vi "Test_WriteValue_InvalidRefnum_Error.vi"(8 "error in (no error)":errorcluster, 11 "TestCase in":refnum<class "TestTerminalSignalingValueBinding.lvclass">) -> (0 "error out":errorcluster, 3 "TestCase out":refnum<class "TestTerminalSignalingValueBinding.lvclass">)   [LabVIEW 2017, in "TestTerminalSignalingValueBinding.lvclass"]
uses:
  TestTerminalSignalingValueBinding.lvclass
  Source/Concrete/TerminalSignalingValueBinding/TerminalSignalingValueBinding.lvclass
  C:/Git/composed-transport/Source/ITransport/ITransport.lvclass
  Source/ITransport/ITransport.lvclass
panel:
  out "Return Error":errorcluster
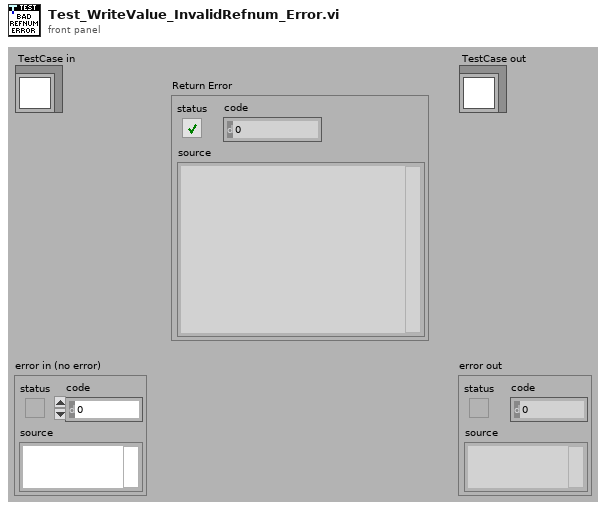
[diagram p1: front panel]
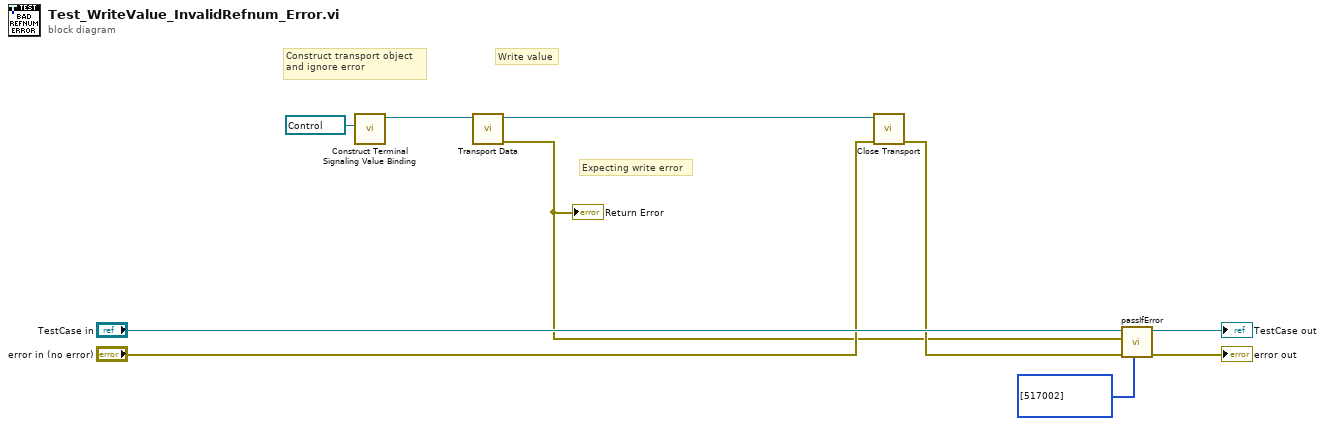
[diagram p0: block diagram]
diagram:
  # "Write value"
  # "Expecting write error"
  # "Construct transport object\nand ignore error"
  n1 = call "Construct Terminal Signaling Value Binding.vi"("Ctl Refnum"=refnum<vi> refnum) -> ("TerminalSignalingValueBinding"=w7:refnum<class "TerminalSignalingValueBinding.lvclass">)  [unwired: 9 in, 1 out]
  n2 = call "Transport Data.vi"("ITransport in"=w7) -> ("error out"=w3:errorcluster, "ITransport out"=w4:refnum<class "TerminalSignalingValueBinding.lvclass">)  [unwired: 9 in]
  "Return Error" <- w3
  n3 = call-dynamic "Close Transport.vi"("error in (no error)"="error in (no error)", "ITransport in"=w4) -> ("error out"=w5:errorcluster)  [unwired: 9 in]
  n4 = call-dynamic "passIfError.vi"("passing error codes (default = any error code)"=i32[] [517002], "error in (no error)"=w5, "error"=w3, "TestCase in"="TestCase in") -> ("error out"=→"error out":errorcluster, "TestCase out"=→"TestCase out":refnum<class "TestTerminalSignalingValueBinding.lvclass">)  [unwired: 6 in]
